vi "Agilis cfg stepSize.vi"(8 "error in (no error)":errorcluster, 9 "Channel parsed command info":T1, 10 "Simulation":T2, 11 "input cluster":refnum<class "AgilisPiezoStage.lvclass">) -> (0 "error out":errorcluster, 1 "new commands":string, 3 "output cluster":refnum<class "AgilisPiezoStage.lvclass">)   [LabVIEW 2013, in "AgilisPiezoStage.lvclass"]
uses:
  AgilisPiezoStage.lvclass
  shared/OnOffTypeDef.ctl
  Shared/Device Driver/channel parsed cmd cluster.ctl
  AgilisPiezoStage.lvclass/AgilisPiezoStage.ctl
  C:/Program Files/Newport/Piezo Motion Control/Newport AG-UC2-UC8 Applet/Samples/LabVIEW 2009/AgilisCmdLib.dll
  Program Files/Newport/Piezo Motion Control/Newport AG-UC2-UC8 Applet/Samples/LabVIEW 2009/AgilisCmdLib.dll
  shared/CompressAndUpdate(Poly)/CompressAndUpdate(Numeric).vi
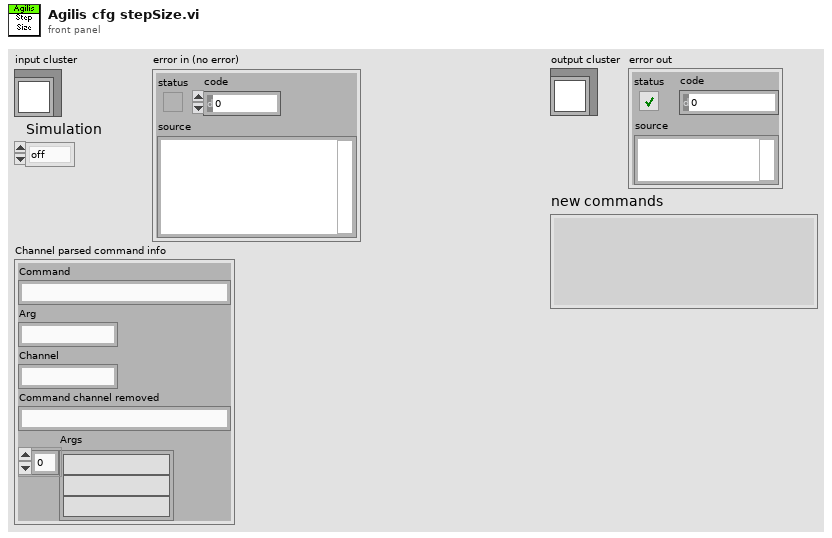
[diagram p1: front panel]
types:
  T1 = typedef "channel parsed cmd cluster.ctl" = cluster{"Command":string, "Arg":string, "Channel":string, "Command channel removed":string, "Args":string[]}
  T2 = typedef "OnOffTypeDef.ctl" = enum16{"off", "on"}
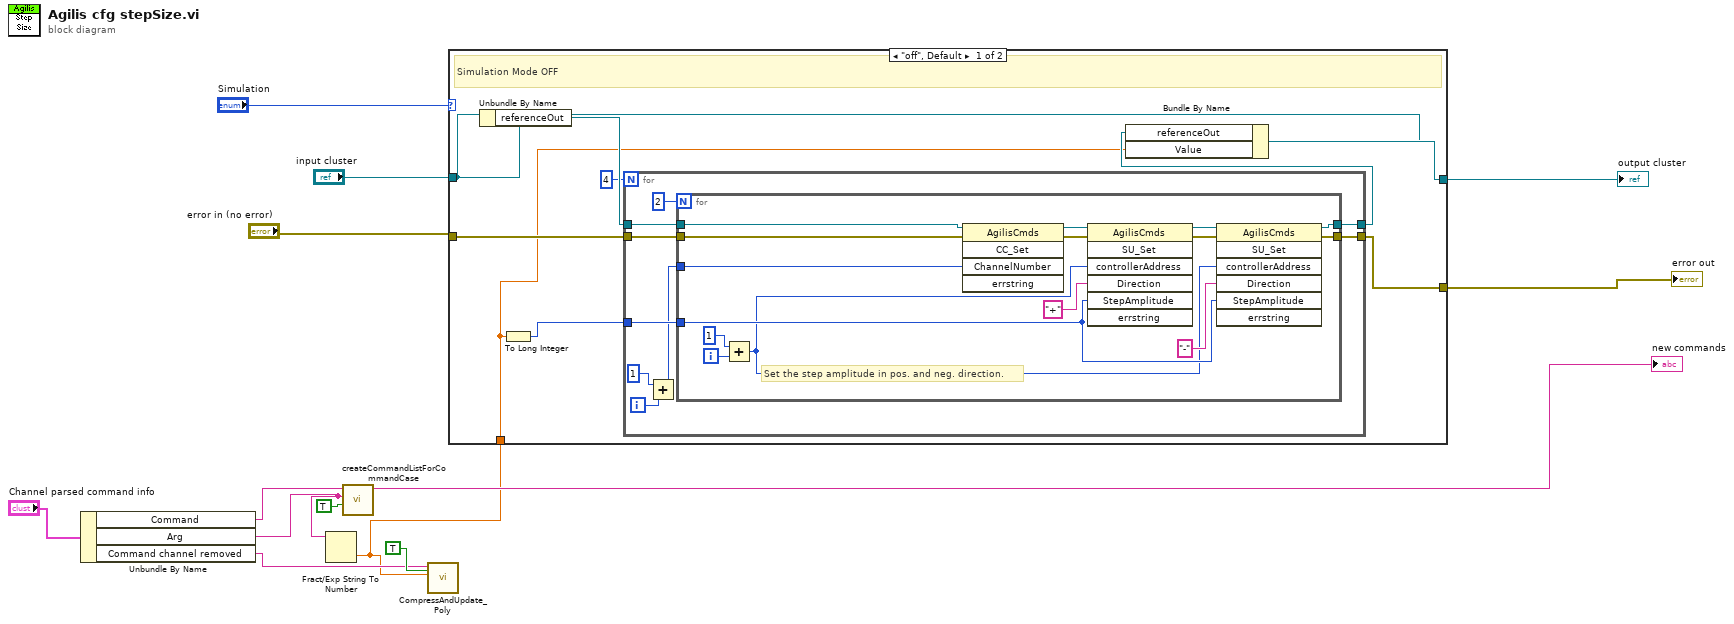
[diagram p0: block diagram]
diagram:
  n1 = Unbundle By Name("Channel parsed command info") -> ("Command"=w10:string, "Arg"=w9:string, "Command channel removed"=w8:string)
  n2 = Fract/Exp String To Number(string=w9) -> (number=w1:dbl)  [unwired: 3 in, 1 out]
  n3 = call "createCommandListForCommandCase.vi"("immediate Check (only once)"=TRUE, "setvalue"=w9, "command"=w10) -> ("new commands"=→"new commands":string)  [unwired: 8 in]
  n4 = call-poly "CompressAndUpdate_Poly.vi"("force CVT update (false)"=TRUE ("force CVT update"), "Numeric"=w1, "command or variable name"=w8) -> ()  [unwired: 8 in, 1 out]
  n5 = case shown="\"off\", Default" "Simulation" {
    tunnel: [w22 w48] -> w4
    tunnel: "input cluster" -> [w21 w48]
    tunnel: "error in (no error)" -> [w19 w47]
    tunnel: [w18 w47] -> w2
    tunnel: w1 -> [w14 _]
    frame "off", Default {
      # "Simulation Mode OFF"
      n6 = Unbundle By Name(w21) -> ("referenceOut"=w20:refnum<k24>)
      n7 = To Long Integer(number=w14) -> (32bit integer=w17:i32)
      n8 = for {
        N: 4 -> [_]
        tunnel: w20 -> [w30]
        tunnel: w19 -> [w29]
        tunnel: [w28] -> w15
        tunnel: [w27] -> w18
        tunnel: w17 -> [w26]
        i -> [w24]
        n9 = Add(x=1, y=w24) -> (x+y=w23:i32)
        n10 = for {
          N: 2 -> [_]
          tunnel: w26 -> [w42]
          tunnel: w30 -> [w39]
          tunnel: w29 -> [w38]
          tunnel: [w35] -> w28
          tunnel: [w34] -> w27
          tunnel: w23 -> [w33]
          i -> [w41]
          # "Set the step amplitude in pos. and neg. direction."
          n11 = Add(x=1, y=w41) -> (x+y=w32:i32)
          n12 = invoke class="AgilisCmds" method="CC_Set"(reference=w39, error in=w38, "ChannelNumber"=w33) -> (reference out=w36:refnum<k24>, error out=w37:errorcluster)  [unwired: 2 in, 3 out]
          n13 = invoke class="AgilisCmds" method="SU_Set"(reference=w36, error in=w37, "controllerAddress"=w32, "Direction"="+", "StepAmplitude"=w42) -> (reference out=w45:refnum<k24>, error out=w44:errorcluster)  [unwired: 2 in, 5 out]
          n14 = invoke class="AgilisCmds" method="SU_Set"(reference=w45, error in=w44, "controllerAddress"=w32, "Direction"="-", "StepAmplitude"=w42) -> (reference out=w35:refnum<k24>, error out=w34:errorcluster)  [unwired: 2 in, 5 out]
        }
      }
      n15 = Bundle By Name(cluster=w21, "referenceOut"=w15, "Value"=w14) -> (w22:refnum<class "AgilisPiezoStage.lvclass">)
    }
    frame "on" {
      # "Simulation Mode ON"
    }
  }
  "output cluster" <- w4
  "error out" <- w2
